vi "Write Session.vi"(8 "error in (no error)":errorcluster, 10 "Session":i32, 11 "UnitTestFramework in":refnum<class "UnitTestFramework.lvclass">) -> (0 "error out":errorcluster, 3 "UnitTestFramework out":refnum<class "UnitTestFramework.lvclass">)   [LabVIEW 2019, in "UnitTestFramework.lvclass"]
uses:
  UnitTestFramework.lvclass
  UnitTestFramework.lvclass/UnitTestFramework.ctl
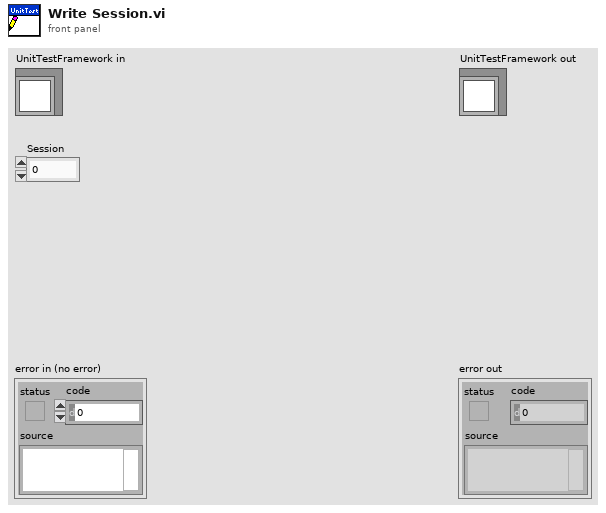
[diagram p1: front panel]
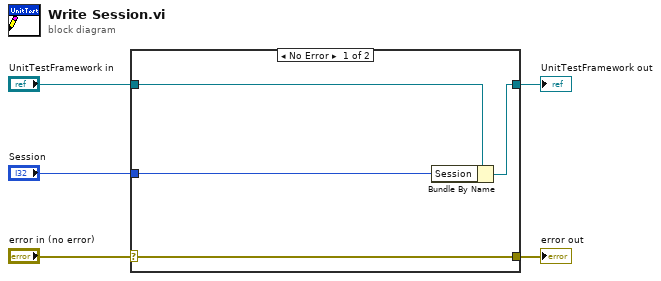
[diagram p0: block diagram]
diagram:
  n1 = case shown="No Error" "error in (no error)" {
    selector: "error in (no error)" -> [w9 w10]
    tunnel: [w9 w10] -> w4
    tunnel: [w7 w11] -> w2
    tunnel: "UnitTestFramework in" -> [w8 w11]
    tunnel: "Session" -> [w6 _]
    frame No Error {
      n2 = Bundle By Name(cluster=w8, "Session"=w6) -> (w7:refnum<class "UnitTestFramework.lvclass">)
    }
    frame Error {
    }
  }
  "error out" <- w4
  "UnitTestFramework out" <- w2
